vi "Write Analog Torque Scale 4.vi"(6 "error in":errorcluster, 8 "MaxRead":i32, 9 "Channel in":u16) -> (0 "error out":errorcluster, 1 "Messages":T1(array[cluster]), 2 "Pass":bool, 3 "Channel out":u16)   [LabVIEW 2023]
uses:
  be2a90bf-c340-472d-9dbd-2edbd756b5ea.vi
  Communication/PCAN2023/PCAN API.lvlib
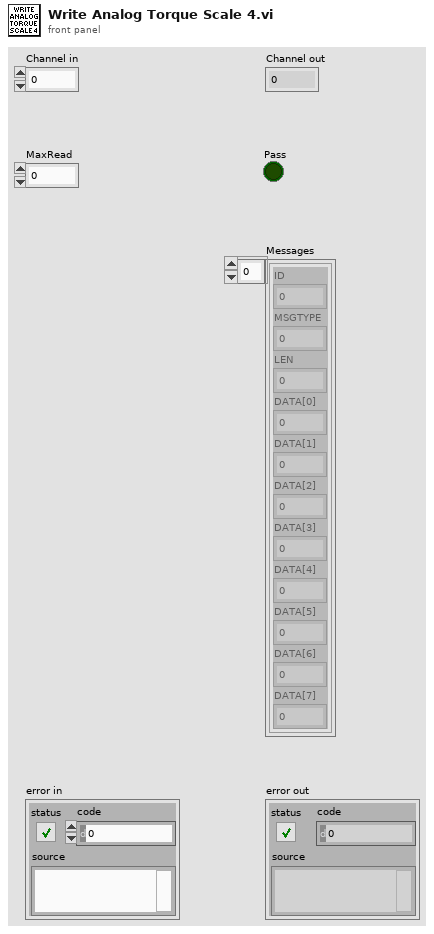
[diagram p1: front panel]
types:
  T1 = cluster{"ID":u32, "MSGTYPE":u8, "LEN":u8, "DATA[0]":u8, "DATA[1]":u8, "DATA[2]":u8, "DATA[3]":u8, "DATA[4]":u8, "DATA[5]":u8, "DATA[6]":u8, "DATA[7]":u8}[]
  T2 = cluster{"ID":u32, "MSGTYPE":u8, "LEN":u8, "DATA[0]":u8, "DATA[1]":u8, "DATA[2]":u8, "DATA[3]":u8, "DATA[4]":u8, "DATA[5]":u8, "DATA[6]":u8, "DATA[7]":u8}
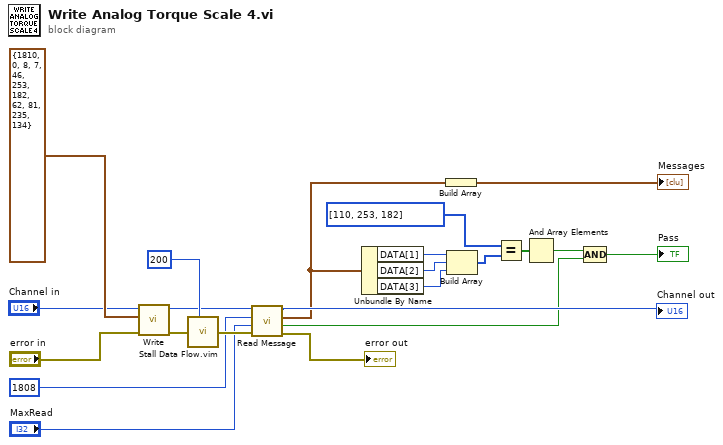
[diagram p0: block diagram]
diagram:
  n1 = call "Write.vi"("error in"="error in", "MessageBuffer"=T2 {"ID"=1810, "MSGTYPE"=0, "LEN"=8, "DATA[0]"=7, "DATA[1]"=46, "DATA[2]"=253, "DATA[3]"=182, "DATA[4]"=62, "DATA[5]"=81, "DATA[6]"=235, "DATA[7]"=134}, "Channel"="Channel in") -> ("error out"=w21:errorcluster, "Channel out"=w8:u16)  [unwired: 5 in, 2 out]
  n2 = call "Stall Data Flow.vim"("value in"=w21, "milliseconds to wait"=u32 200) -> ("value out"=w7:errorcluster)  [unwired: 1 out]
  n3 = call "Read Message.vi"("error in"=w7, "MaxRead"="MaxRead", "ID"=u32 1808, "Channel in"=w8) -> ("error out"=→"error out":errorcluster, "Passed"=w2:bool, "Last Message"=w3:T2, "Channel out"=→"Channel out":u16)  [unwired: 3 in, 1 out]
  n4 = Unbundle By Name(w3) -> ("DATA[1]"=w14:u8, "DATA[2]"=w13:u8, "DATA[3]"=w12:u8)
  n5 = Build Array(w3) -> (→"Messages":T1)
  n6 = Build Array(w14, w13, w12) -> (w11:u8[])
  n7 = Equal?(x=u8[] [110, 253, 182], y=w11) -> (x = y?=w17:bool[])
  n8 = And Array Elements(Boolean array=w17) -> (logical AND=w10:bool)
  n9 = Compound Arithmetic op=AND(w10, w2) -> (→"Pass":bool)
